vi "read shared variable.vi"(11 "shared variable refnum in":string) -> (3 "data out":i32)   [LabVIEW 2020, in "GaiaSVEReader.lvclass"]
uses:
  GaiaSVEReader.lvclass
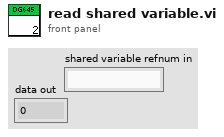
[diagram p1: front panel]
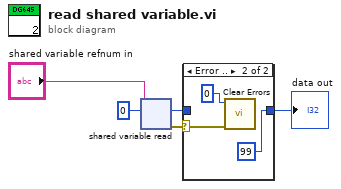
[diagram p0: block diagram]
diagram:
  n1 = shared-variable-read("shared variable refnum in", 0) -> (w4:errorcluster, w3:i32)  [unwired: 1 in, 2 out]
  n2 = case shown="Error .." w4 {
    selector: w4 -> [_ w8]
    tunnel: w3 -> [w6 _]
    tunnel: [w6 99] -> w5
    frame No Error {
    }
    frame Error {
      n3 = call <vilib>:"Clear Errors.vi"("error in (no error)"=w8, "specific error code to clear (0: all)"=0) -> ()  [unwired: 4 in, 2 out]
    }
  }
  "data out" <- w5
